vi "Result_Test.vi"(8 "error in (no error)":errorcluster caption="entrée d'erreur (pas d'erreur)", 11 "Delay en entrée":refnum<class "Nodon_Scan_SN.lvclass">) -> (0 "error out":errorcluster caption="sortie d'erreur", 3 "Delay en sortie":refnum<class "Nodon_Scan_SN.lvclass">)   [LabVIEW 2020, in "Library Test.lvlib" / "Nodon_Scan_SN.lvclass"]
uses:
  Nodon_Scan_SN.lvclass
  C:/Users/ngarcin/OneDrive - Altyor/Standard TB/Class/Test/Test (Default)/Test (Default).lvclass
  Test_Without_Instr/Test_Without_Inst.lvclass
  Nodon_Scan_SN.lvclass/Nodon_Scan_SN.ctl
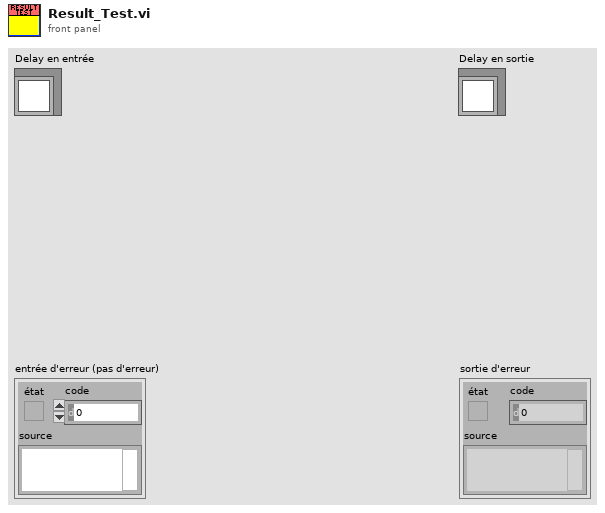
[diagram p1: front panel]
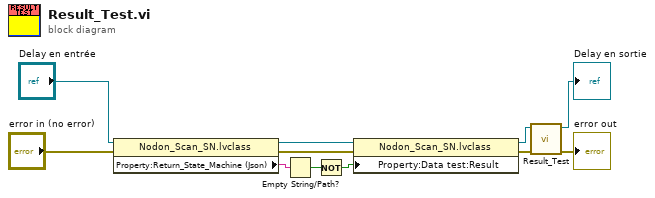
[diagram p0: block diagram]
diagram:
  n1 = property class="Nodon_Scan_SN.lvclass"(reference="Delay en entrée", error in="error in (no error)") -> (reference out=w7:refnum<class "Nodon_Scan_SN.lvclass">, error out=w2:errorcluster, "Property:Return_State_Machine (Json)"=w5:string)
  n2 = Empty String/Path?(string/path=w5) -> (empty?=w4:bool)
  n3 = Not(x=w4) -> (.not. x?=w3:bool)
  n4 = property class="Nodon_Scan_SN.lvclass"(reference=w7, error in=w2, "Property:Data test:Result"=w3) -> (reference out=w6:refnum<class "Nodon_Scan_SN.lvclass">, error out=w1:errorcluster)
  n5 = call-parent "Result_Test.vi"("error in (no error)"=w1, "Test_Without_Inst en entrée"=w6) -> ("error out"=→"error out":errorcluster, "Test_Without_Inst en sortie"=→"Delay en sortie":refnum<class "Nodon_Scan_SN.lvclass">)  [unwired: 8 in]
